vi "Extract VI Strings.vi"(0 "SET VI in":refnum<class "VI Data.lvclass">, 1 "VI Ref in":refnum<vi>, 3 "error in (no error)":errorcluster) -> (7 "SET VI out":refnum<class "VI Data.lvclass">, 8 "VI Ref out":refnum<vi>, 10 "error out":errorcluster)   [LabVIEW 2013, in "SET Project Data.lvlib" / "VI Data.lvclass"]
uses:
  VI Data.lvclass
  VI Data.lvclass/VI Data.ctl
  Control Classes/GObject/GObject.lvclass
panel:
  # "Extract strings that are not GObjects:\n- FPTitle"
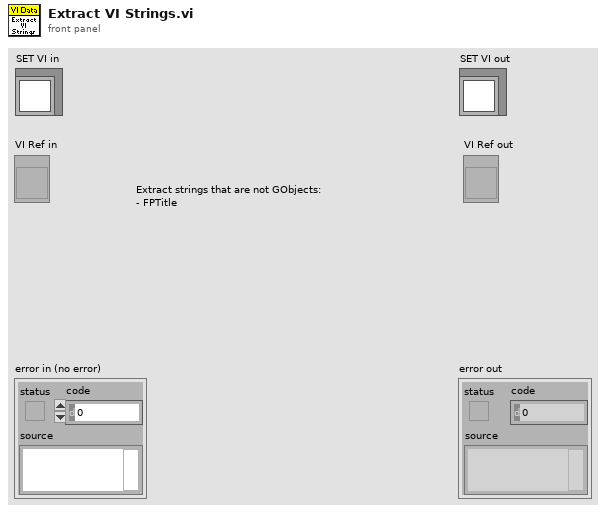
[diagram p1: front panel]
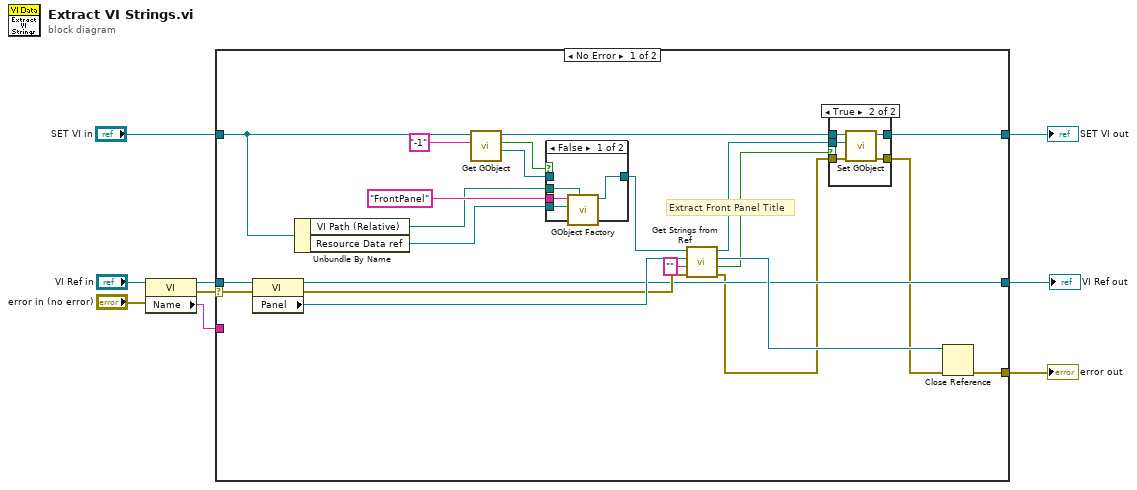
[diagram p0: block diagram]
diagram:
  n1 = property class="VI"(reference="VI Ref in", error in="error in (no error)") -> (reference out=w5:refnum<vi>, error out=w3:errorcluster, "Name"=w4:string)
  n2 = case shown="No Error" w3 {
    selector: w3 -> [w30 w46]
    tunnel: [w27 w46] -> w9
    tunnel: [w23 w45] -> w7
    tunnel: "SET VI in" -> [w22 w45]
    tunnel: w4 -> [_ _]
    tunnel: w5 -> [w31 w44]
    tunnel: [w25 w44] -> w1
    frame No Error {
      # "Extract Front Panel Title"
      n3 = property class="VI"(reference=w31, error in=w30) -> (reference out=w25:refnum<vi>, error out=w28:errorcluster, "Panel"=w29:refnum<vi>)
      n4 = Unbundle By Name(w22) -> ("VI Path (Relative)"=w16:path, "Resource Data ref"=w15:refnum<data-value>)
      n5 = call-dynamic "Get GObject.vi"("GObject UID"="-1", "VI Data in"=w22) -> ("GObject"=w19:refnum<class "GObject.lvclass">, "found"=w20:bool, "VI Data out"=w18:refnum<class "VI Data.lvclass">)  [unwired: 6 in, 1 out]
      n6 = case shown="False" w20 {
        tunnel: w19 -> [_ w43]
        tunnel: "FrontPanel" ("ClassName") -> [w42 _]
        tunnel: w16 -> [w41 _]
        tunnel: w15 -> [w40 _]
        tunnel: [w39 w43] -> w14
        frame False {
          n7 = call "GObject Factory.vi"("Owning VI"=w41, "LangFile ref"=w40, "ClassName"=w42) -> ("GObject"=w39:refnum<class "GObject.lvclass">)  [unwired: 8 in]
        }
        frame True {
        }
      }
      n8 = call-dynamic "Get Strings from Ref.vi"("error in (no error)"=w28, "Label Prefix"="", "GObj Refnum in"=w29, "GObject in"=w14) -> ("error out"=w11:errorcluster, "Valid?"=w13:bool, "GObj Refnum out"=w26:refnum<vi>, "GObject out"=w12:refnum<class "GObject.lvclass">)  [unwired: 3 in, 1 out]
      n9 = case shown="True" w13 {
        tunnel: [w33 w38] -> w23
        tunnel: w18 -> [w33 w37]
        tunnel: w12 -> [_ w36]
        tunnel: w11 -> [w32 w35]
        tunnel: [w32 w34] -> w10
        frame False {
        }
        frame True {
          n10 = call "Set GObject.vi"("error in (no error)"=w35, "GObject.lvclass"=w36, "VI Data in"=w37) -> ("error out"=w34:errorcluster, "VI Data out"=w38:refnum<class "VI Data.lvclass">)  [unwired: 6 in, 1 out]
        }
      }
      n11 = Close Reference(reference=w26, error in (no error)=w10) -> (error out=w27:errorcluster)
    }
    frame Error {
    }
  }
  "error out" <- w9
  "SET VI out" <- w7
  "VI Ref out" <- w1
